vi "Get associated LV error.vi"(11 "IErrorHandler in":refnum<class "AbortHandler JSON.lvclass">) -> (2 "Associated LabVIEW Error":errorcluster, 3 "IErrorHandler out":refnum<class "AbortHandler JSON.lvclass">)   [LabVIEW 2020, in "wamplv.lvlib" / "AbortHandler JSON.lvclass"]
uses:
  AbortHandler JSON.lvclass
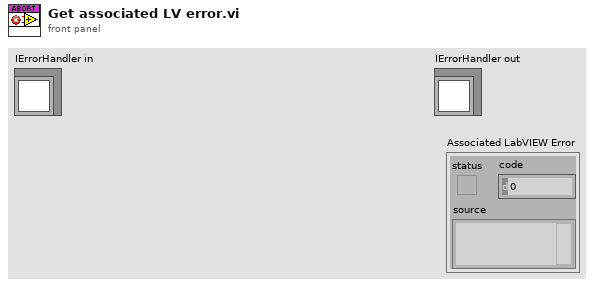
[diagram p1: front panel]
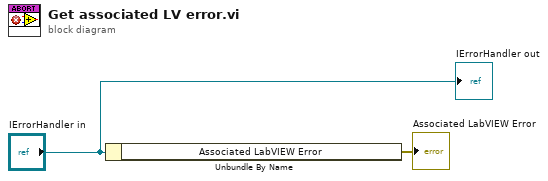
[diagram p0: block diagram]
diagram:
  n1 = Unbundle By Name("IErrorHandler in") -> ("Associated LabVIEW Error"=→"Associated LabVIEW Error":errorcluster)
  "IErrorHandler out" <- "IErrorHandler in"
